vi "settingsLow.vi"(8 "error in (no error)":errorcluster, 11 "reference in":refnum<class "Project Panels.lvclass">) -> (0 "error out":errorcluster, 3 "reference out":refnum<class "Project Panels.lvclass">)   [LabVIEW 2015, in "Project Panels.lvclass"]
uses:
  Project Panels.lvclass
  GUI Controller_llb/state.ctl
  GUI Controller_llb/GUI Controller.lvclass
  SYS/File Controller_llb/File Controller.lvclass
panel:
  out "Title":string
  in  "not_tracking":bool caption="Notification"
  in  "not_items":bool caption="Notification"
  in  "Tab Control":T1(tab)
  in  "K5:":path
  in  "BB-PFT":path
  in  "RMR-ICU:":path
  in  "Pea Pod:":path
  in  "Bod Pod:":path
  in  "RMR:":path
  in  "CPET:":path
  in  "Fitmate:":path
  in  "K4b2:":path
  in  "K5:2":path caption="K5:"
  in  "BB-PFT 2":path caption="Body Box - PFT:"
  in  "RMR-ICU 2":path caption="RMR-ICU:"
  in  "Pea Pod: 2":path caption="Pea Pod:"
  in  "Bod Pod: 2":path caption="Bod Pod:"
  in  "RMR: 2":path caption="RMR:"
  in  "CPET: 2":path caption="CPET:"
  in  "Fitmate: 2":path caption="Fitmate:"
  in  "K4b2: 2":path caption="K4b2:"
  in  "PartsTracking:":path
  in  "Items:":path
  in  "Products:":path
  out "StatusBar":string
  in  "Save Button":bool
  in  "Stop Button":bool
  # "Excel Files paths:"
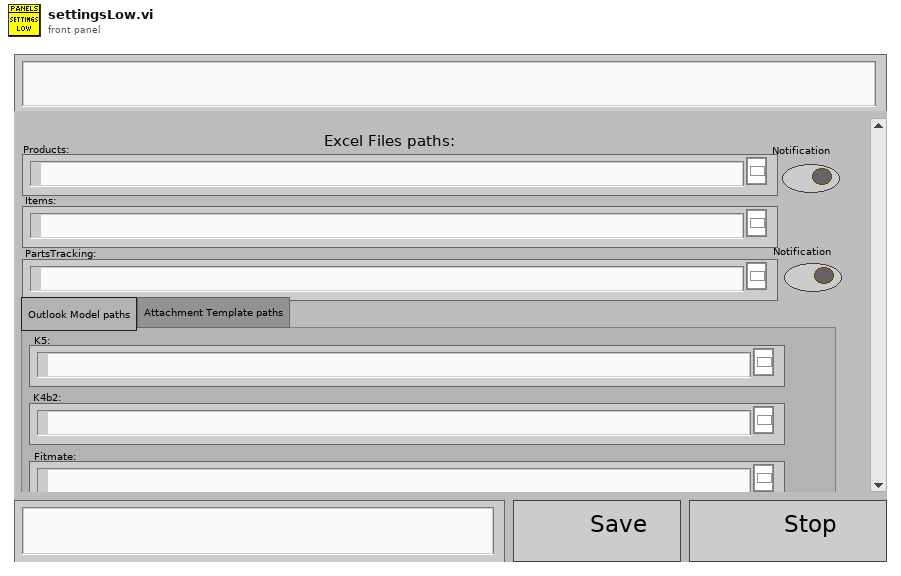
[diagram p1: front panel]
types:
  T1 = enum32{"Outlook Model paths", "Attachment Template paths"}
  T2 = typedef "GUI Controller.lvclass/state.ctl" = enum16{"initiate", "checkNotificationItems", "checkNotificationTracking", "operate", "updateFromFile", "stop"}
  T3 = typedef "Project Panels.lvclass/ObjectAttributesRef.ctl" = refnum<data-value>
  T4 = typedef "Project Panels.lvclass/ObjectAttributes.ctl" = cluster{"MyAttribute":dbl, "device_controller_ref":refnum<class "Devices Controller.lvclass">, "file_controller_ref":refnum<class "File Controller.lvclass">, "item_controller_ref":refnum<class "Items Controller.lvclass">, "item_tables":cluster{"checkIN":string[][], "checkOUT":string[][], "storage":string[][]}, "quickbook_table":cluster{"notes":string[][]}, "notification_controller_ref":refnum<class "Notification Controller.lvclass">, "partstracking_controller_ref":refnum<class "PartsTracking Controller.lvclass">, "product_tables":cluster{"k4b2":string[][], "fitmate":string[][], "RMR":string[][], "CPET":string[][], "BP":string[][], "PP":string[][], "k5":string[][], "bb-pft":string[][]}, "rowsColour":u32[], "low_resolution?":bool}
  T5 = cluster{"filePaths":path[], "outlookTemplatePaths":path[], "attachmentTemplatePaths":path[]}
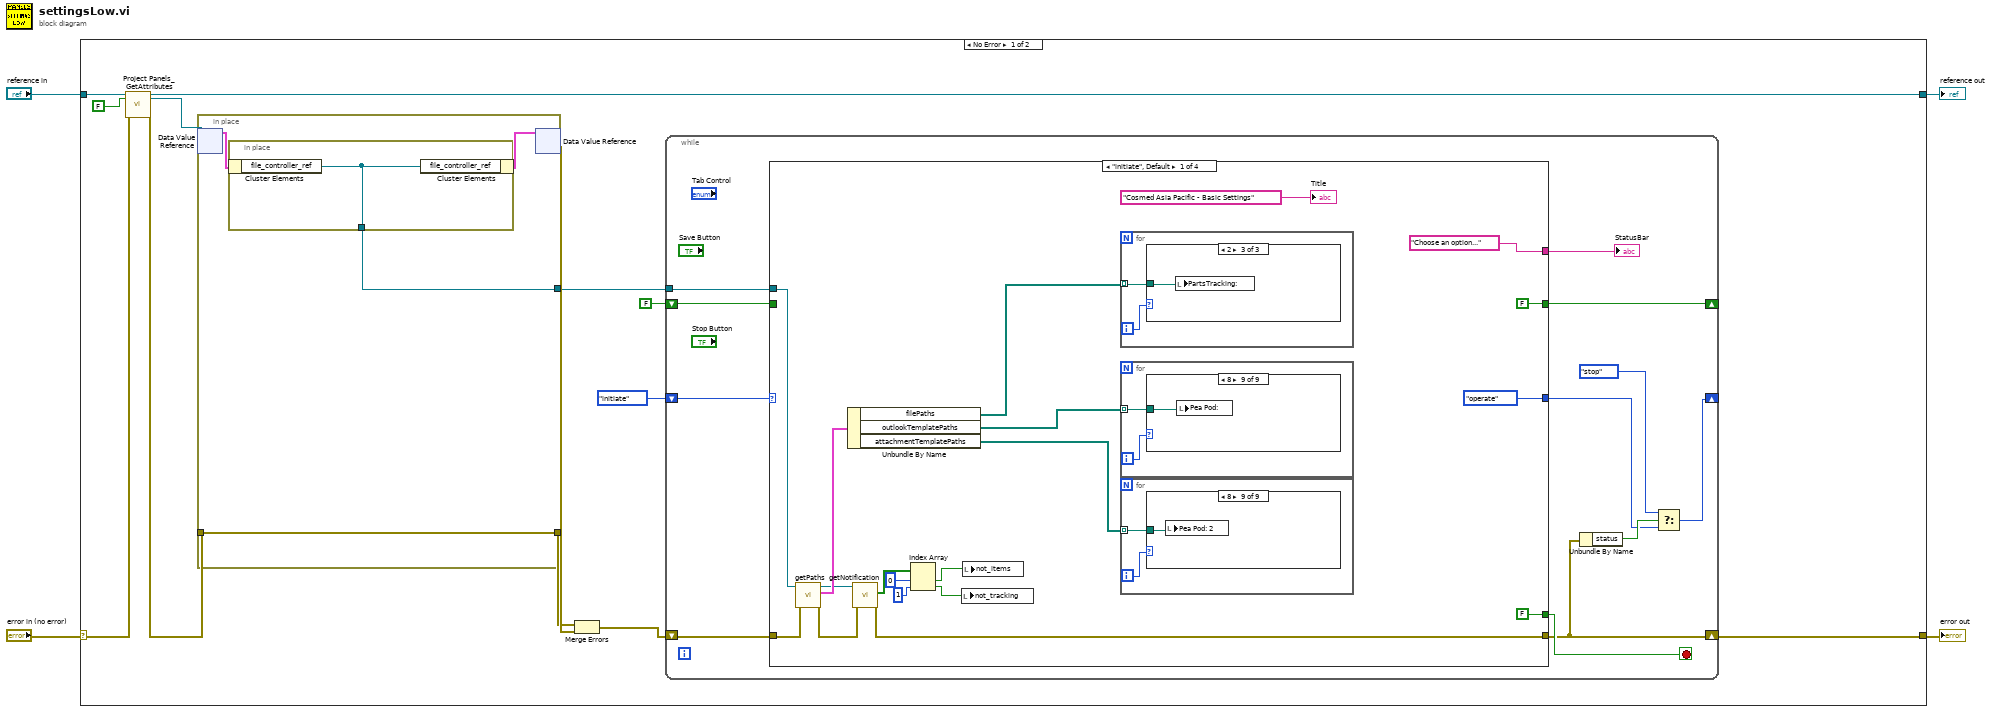
[diagram p0: block diagram]
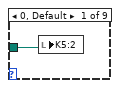
[diagram p2: hidden frame]
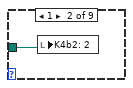
[diagram p3: hidden frame]
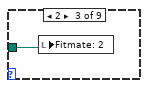
[diagram p4: hidden frame]
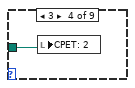
[diagram p5: hidden frame]
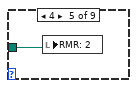
[diagram p6: hidden frame]
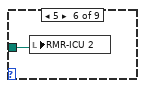
[diagram p7: hidden frame]
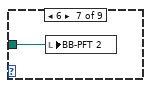
[diagram p8: hidden frame]
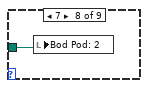
[diagram p9: hidden frame]
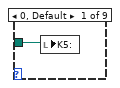
[diagram p10: hidden frame]
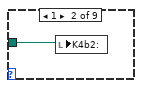
[diagram p11: hidden frame]
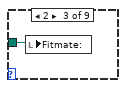
[diagram p12: hidden frame]
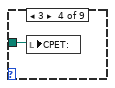
[diagram p13: hidden frame]
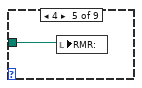
[diagram p14: hidden frame]
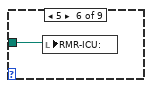
[diagram p15: hidden frame]
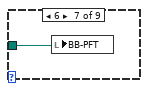
[diagram p16: hidden frame]
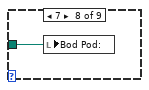
[diagram p17: hidden frame]
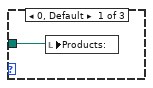
[diagram p18: hidden frame]
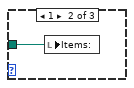
[diagram p19: hidden frame]
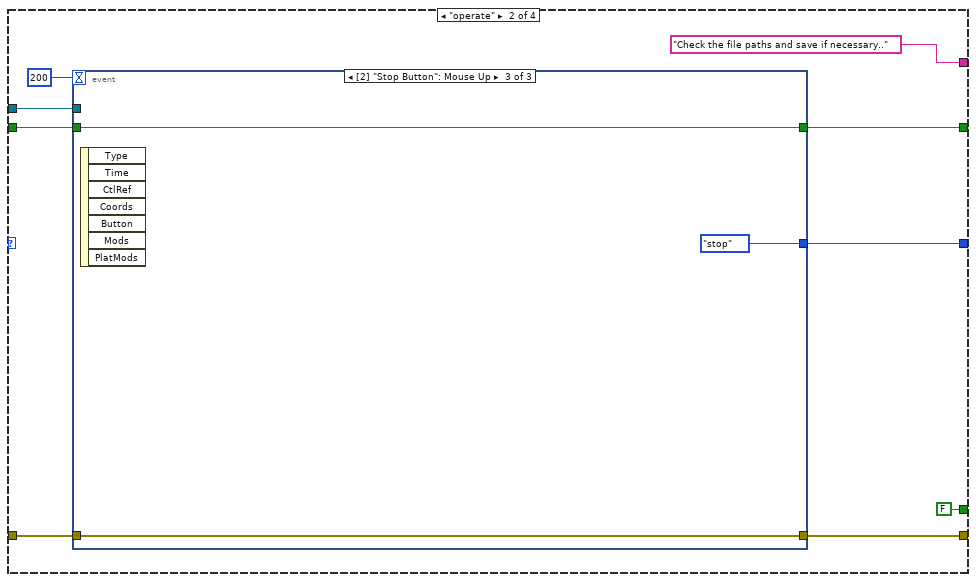
[diagram p20: hidden frame]
diagram:
  n1 = case shown="No Error" "error in (no error)" {
    selector: "error in (no error)" -> [w13 w171]
    tunnel: [w6 w171] -> w3
    tunnel: [w11 w170] -> w1
    tunnel: "reference in" -> [w15 w170]
    frame No Error {
      n2 = call "Project Panels_GetAttributes.vi"("reference in"=w15, "return data? (T)"=FALSE, "error in (no error)"=w13) -> ("reference out"=w11:refnum<class "Project Panels.lvclass">, "attributes ref"=w10:T3, "error out"=w12:errorcluster)  [unwired: 13 in, 1 out]
      n3 = in-place {
        in-place-border: w12 -> [w166]
        in-place-border: [w166] -> w16
        in-place-border: [w165] -> w7
        n4 = in-place-dvr #1(w10) -> (w167:T4)  [unwired: 1 out]
        n5 = in-place {
          in-place-border: [w169] -> w165
          n6 = in-place-cluster #2(w167) -> ("file_controller_ref"=w169:refnum<class "File Controller.lvclass">)
          n7 = in-place-cluster #2("file_controller_ref"=w169) -> (w168:T4)
        }
        n8 = in-place-dvr #1(w168) -> (w17:errorcluster)  [unwired: 1 out]
      }
      n9 = Merge Errors(w16, w17) -> (w9:errorcluster)
      n10 = while {
        shift-right: [w23] -> _
        shift-left: state."initiate" ("state") -> [w28]
        shift-right: [w25] -> w6
        shift-left: w9 -> [w29]
        tunnel: w7 -> [w22]
        shift-right: [w19] -> _
        shift-left: FALSE -> [w18]
        stop <- w26 stop-if-true
        n11 = case shown="\"initiate\", Default" w28 {
          tunnel: w29 -> [w43 w82 w112 w139]
          tunnel: [w35 w81 w117 w138] -> w25
          tunnel: [state."operate" ("state") w78 state."operate" ("state") w137] -> w21
          tunnel: ["Choose an option..." ("Title") "Check the file paths and save if necessary.." ("Title") "Saving....." ("Title") "Stopped..." ("Title")] -> w27
          tunnel: [FALSE FALSE FALSE ("Save") w136] -> w26
          tunnel: w22 -> [w44 w79 w118 _]
          tunnel: [FALSE w77 TRUE FALSE] -> w19
          tunnel: w18 -> [_ w76 _ w140]
          frame "initiate", Default {
            n12 = call "getPaths.vi"("error in (no error)"=w43, "reference in"=w44) -> ("error out"=w36:errorcluster, "paths"=w42:T5, "reference out"=w37:refnum<class "File Controller.lvclass">)  [unwired: 7 in]
            n13 = Unbundle By Name(w42) -> ("filePaths"=w41:path[], "outlookTemplatePaths"=w40:path[], "attachmentTemplatePaths"=w39:path[])
            n14 = call "getNotification.vi"("error in (no error)"=w36, "reference in"=w37) -> ("error out"=w35:errorcluster, "not_setting"=w34:bool[])  [unwired: 7 in, 1 out]
            n15 = Index Array(array=w34, index #1=0 ("index"), index #2=1 ("index")) -> (element #1=w31:bool, element #2=w30:bool)
            n16 = local write "not_tracking"(w30) -> ()
            n17 = local write "not_items"(w31) -> ()
            n18 = for {
              tunnel: w41 -> [w71] mode=indexing
              i -> [w72]
              n19 = case shown="2" w72 {
                tunnel: w71 -> [w73 w74 w75]
                frame 0, Default {
                  n20 = local write "Products:"(w73) -> ()
                }
                frame 1 {
                  n21 = local write "Items:"(w74) -> ()
                }
                frame 2 {
                  n22 = local write "PartsTracking:"(w75) -> ()
                }
              }
            }
            n23 = for {
              tunnel: w40 -> [w60] mode=indexing
              i -> [w61]
              n24 = case shown="8" w61 {
                tunnel: w60 -> [w62 w63 w64 w65 w66 w67 w68 w69 w70]
                frame 0, Default {
                  n25 = local write "K5:"(w62) -> ()
                }
                frame 1 {
                  n26 = local write "K4b2:"(w63) -> ()
                }
                frame 2 {
                  n27 = local write "Fitmate:"(w64) -> ()
                }
                frame 3 {
                  n28 = local write "CPET:"(w65) -> ()
                }
                frame 4 {
                  n29 = local write "RMR:"(w66) -> ()
                }
                frame 5 {
                  n30 = local write "RMR-ICU:"(w67) -> ()
                }
                frame 6 {
                  n31 = local write "BB-PFT"(w68) -> ()
                }
                frame 7 {
                  n32 = local write "Bod Pod:"(w69) -> ()
                }
                frame 8 {
                  n33 = local write "Pea Pod:"(w70) -> ()
                }
              }
            }
            n34 = for {
              tunnel: w39 -> [w49] mode=indexing
              i -> [w50]
              n35 = case shown="8" w50 {
                tunnel: w49 -> [w51 w52 w53 w54 w55 w56 w57 w58 w59]
                frame 0, Default {
                  n36 = local write "K5:2"(w51) -> ()
                }
                frame 1 {
                  n37 = local write "K4b2: 2"(w52) -> ()
                }
                frame 2 {
                  n38 = local write "Fitmate: 2"(w53) -> ()
                }
                frame 3 {
                  n39 = local write "CPET: 2"(w54) -> ()
                }
                frame 4 {
                  n40 = local write "RMR: 2"(w55) -> ()
                }
                frame 5 {
                  n41 = local write "RMR-ICU 2"(w56) -> ()
                }
                frame 6 {
                  n42 = local write "BB-PFT 2"(w57) -> ()
                }
                frame 7 {
                  n43 = local write "Bod Pod: 2"(w58) -> ()
                }
                frame 8 {
                  n44 = local write "Pea Pod: 2"(w59) -> ()
                }
              }
            }
            "Title" <- "Cosmed Asia Pacific - Basic Settings" ("Title")
          }
          frame "operate" {
            n45 = event shown="[2] \"Stop Button\": Mouse Up" {
              selector: _ -> [_ _ _]
              dyn-events: _ -> [_ _ _]
              timeout: 200 -> [_ _ _]
              tunnel: w82 -> [w86 w88 w91]
              tunnel: [w86 w88 w91] -> w81
              tunnel: w79 -> [_ _ _]
              tunnel: [state."operate" ("state") state."updateFromFile" ("state") state."stop" ("state")] -> w78
              tunnel: [w85 FALSE w92] -> w77
              tunnel: w76 -> [w85 _ w92]
              event Timeout {
                n46 = event-data() -> ()  [unwired: 1 in, 2 out]
              }
              event "Save Button": Mouse Up {
                n47 = event-data() -> ()  [unwired: 1 in, 7 out]
              }
              event "Stop Button": Mouse Up {
                n48 = event-data() -> ()  [unwired: 1 in, 7 out]
              }
            }
          }
          frame "updateFromFile" {
            n49 = flat-sequence {
              tunnel: w112 -> [w135]
              tunnel: [w135] -> w111
              frame #0 {
                n50 = local write "StatusBar"("Saving..." ("StatusBar")) -> ()
                n51 = Wait (ms)(milliseconds to wait=u32 1000) -> ()  [unwired: 1 out]
              }
            }
            n52 = Build Array("Products:", "Items:", "PartsTracking:") -> (w119:path[])
            n53 = Build Array("K5:", "K4b2:", "Fitmate:", "CPET:", "RMR:", "RMR-ICU:", "BB-PFT", "Bod Pod:", "Pea Pod:") -> (w120:path[])
            n54 = Build Array("K5:2", "K4b2: 2", "Fitmate: 2", "CPET: 2", "RMR: 2", "RMR-ICU 2", "BB-PFT 2", "Bod Pod: 2", "Pea Pod: 2") -> (w121:path[])
            n55 = call "setPaths.vi"("reference in"=w118, "filePaths"=w119, "outlookTemplatePaths"=w120, "attachmentTemplatePaths"=w121, "error in (no error)"=w111) -> ("reference out"=w107:refnum<class "File Controller.lvclass">, "error out"=w105:errorcluster)  [unwired: 9 in]
            n56 = Build Array("not_items", "not_tracking") -> (w108:bool[])
            n57 = call "setNotificationSettings.vi"("error in (no error)"=w105, "not_settings"=w108, "reference in"=w107) -> ("error out"=w104:errorcluster, "reference out"=w106:refnum<class "File Controller.lvclass">)  [unwired: 7 in]
            n58 = call "saveData.vi"("error in (no error)"=w104, "reference in"=w106) -> ("error out"=w117:errorcluster)  [unwired: 8 in, 1 out]
          }
          frame "stop" {
            n59 = Unbundle By Name(w139) -> ("status"=w142:bool)
            n60 = case shown="False" w142 {
              tunnel: w139 -> [w150 w161]
              tunnel: w140 -> [w151 _]
              tunnel: [w149 w161] -> w138
              tunnel: [w146 state."initiate" ("state")] -> w137
              tunnel: [w144 TRUE ("Save")] -> w136
              frame False {
                n61 = case shown="False" w151 {
                  tunnel: w150 -> [w156 w157]
                  tunnel: [w156 w157] -> w149
                  tunnel: [w154 FALSE ("Save")] -> w145
                  frame False {
                    n62 = Two Button Dialog(message="The panel will be closed without saving the data. Do you want to save the data?", 1:"Not Save" ("F button name (\"Cancel\")"), 2:"Save" ("T button name (\"OK\")")) -> (T button?=w154:bool)
                  }
                  frame True {
                  }
                }
                n63 = Not(x=w145) -> (.not. x?=w144:bool)
                n64 = Select(t=state."updateFromFile" ("state"), s=w145, f=state."stop" ("state")) -> (s? t:f=w146:T2)
              }
              frame True {
                n65 = Unbundle By Name(w161) -> ("source"=w162:string)
                n66 = Concatenate Strings("An Error occur: " ("message"), w162) -> (w164:string)
                n67 = One Button Dialog(message=w164) -> ()  [unwired: 1 in, 1 out]
              }
            }
          }
        }
        "StatusBar" <- w27
        n68 = Unbundle By Name(w25) -> ("status"=w24:bool)
        n69 = Select(t=state."stop", s=w24, f=w21) -> (s? t:f=w23:T2)
      }
    }
    frame Error {
    }
  }
  "error out" <- w3
  "reference out" <- w1
